vi "Test Set Myltiple Symbols.vi"(8 "error in (no error)":errorcluster, 11 "Test Case In":refnum<class "Conditional Disabled Configurator Test.lvclass">) -> (0 "error out":errorcluster, 3 "Test Case Out":refnum<class "Conditional Disabled Configurator Test.lvclass">)   [LabVIEW 2020, in "Conditional Disabled Configurator Test.lvclass"]
uses:
  Conditional Disabled Configurator Test.lvclass
  Conditional Disabled Configurator Test.lvclass/Conditional Disabled Configurator Test.ctl
  01074fa8-ee8a-411d-bc8b-fc92c4f90959.vi
  source/Conditional Disabled Configurator/Conditional Disabled Configurator.lvclass
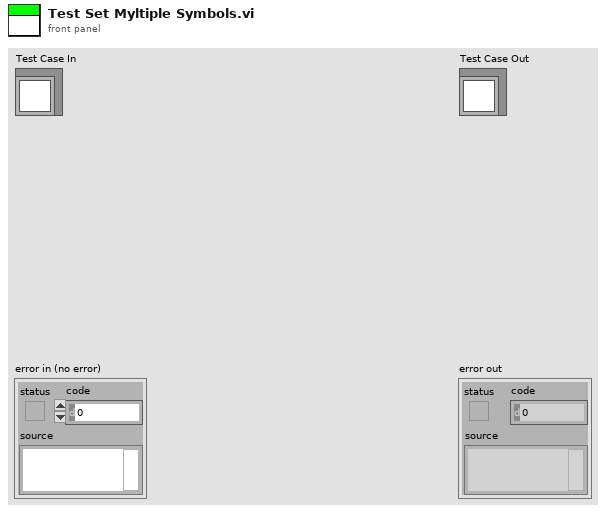
[diagram p1: front panel]
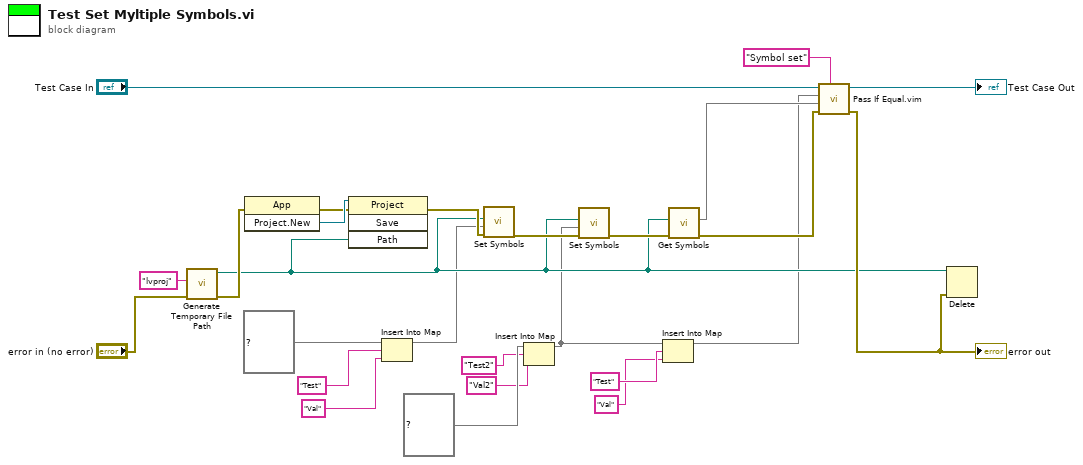
[diagram p0: block diagram]
diagram:
  n1 = call <vilib>:"Generate Temporary File Path.vi"("error in (no error)"="error in (no error)", "Temporary File Extension (tmp)"="lvproj") -> ("error out"=w22:errorcluster, "Unique Temporary File Path"=w6:path)  [unwired: 8 in]
  n2 = invoke class="App" method="Project.New"(error in=w22) -> (error out=w20:errorcluster, "Project:New"=w21:refnum<vi>)  [unwired: 2 in, 1 out]
  n3 = invoke class="Project" method="Save"(reference=w21, error in=w20, "Path"=w6) -> (error out=w19:errorcluster)  [unwired: 1 in, 3 out]
  n4 = Insert Into Map(map in=map{string, string} {} ("Symbols"), key="Test", value="Val") -> (map out=w2:map{string, string})  [unwired: 2 out]
  n5 = call "Set Symbols.vi"("error in (no error)"=w19, "Symbols"=w2, "Project Path"=w6) -> ("error out"=w11:errorcluster)  [unwired: 8 in]
  n6 = Insert Into Map(map in=map{string, string} {} ("Symbols"), key="Test2", value="Val2") -> (map out=w5:map{string, string})  [unwired: 2 out]
  n7 = call "Set Symbols.vi"("error in (no error)"=w11, "Symbols"=w5, "Project Path"=w6) -> ("error out"=w10:errorcluster)  [unwired: 8 in]
  n8 = Insert Into Map(map in=w5, key="Test", value="Val") -> (map out=w1:map{string, string})  [unwired: 2 out]
  n9 = call "Get Symbols.vi"("error in (no error)"=w10, "Project Path"=w6) -> ("error out"=w14:errorcluster, "Symbols"=w15:map{string, string})  [unwired: 8 in]
  n10 = call "Pass If Equal.vim"("Description"="Symbol set", "error in (no error)"=w14, "Actual"=w15, "Expected"=w1, "LUnit Test Case In"="Test Case In") -> ("error out"=w12:errorcluster, "LUnit Test Case Out"=→"Test Case Out":refnum<class "Conditional Disabled Configurator Test.lvclass">)  [unwired: 5 in]
  "error out" <- w12
  n11 = Delete(path (use dialog)=w6, error in=w12) -> ()  [unwired: 3 in, 3 out]
